vi "HEWH Write Standard Tests.vi"(8 "Error In":errorcluster, 11 "24HR Test - Standard":T1[](array[typedef])=[{"Sequence #"=1.0, "Cycles"=1, "Mode Setting"="", "Flow Rate (GPM)"=3.0, "Temperature (F)"=58.0, "Reset Timer"=FALSE, "Use Temp Decline Method"=FALSE, "Terminate Condition"=enum."C9-Do Nothing", "Condition Value #1"=0.0, "UE"=FALSE, "LE"=FALSE, "Comp"=FALSE, "Fan"=FALSE, "Test End Time (Sec)"=0.0, "Purge Until Cutout"=FALSE, "Start Conditions"=enum."Heat Source Cutout", "Condition Value #2"=0.0, "Remove Power"=FALSE, "Time"=82800.0, "Check Special Cond."=enum."SC1-Do Nothing", "Condition#"=enum."N/A", "Draw Flags"=enum."N/A", "Data Processing Delay (FHD 15sec, UEF 5 Sec)"=5.0, "Test Complete"=FALSE}, {"Sequence #"=2.0, "Cycles"=1, "Mode Setting"="", "Flow Rate (GPM)"=3.0, "Temperature (F)"=58.0, "Reset Timer"=TRUE, "Use Temp Decline Method"=TRUE, "Terminate Condition"=enum."C1-Terminate Draw @ Gallon Mark", "Condition Value #1"=10.72, "UE"=FALSE, "LE"=FALSE, "Comp"=FALSE, "Fan"=FALSE, "Test End Time (Sec)"=0.0, "Purge Until Cutout"=FALSE, "Start Conditions"=enum."At Time (Seconds)", "Condition Value #2"=0.0, "Remove Power"=FALSE, "Time"=82800.0, "Check Special Cond."=enum."SC1-Do Nothing", "Condition#"=enum."N/A", "Draw Flags"=enum."N/A", "Data Processing Delay (FHD 15sec, UEF 5 Sec)"=5.0, "Test Complete"=FALSE}, {"Sequence #"=3.0, "Cycles"=1, "Mode Setting"="", "Flow Rate (GPM)"=3.0, "Temperature (F)"=58.0, "Reset Timer"=FALSE, "Use Temp Decline Method"=FALSE, "Terminate Condition"=enum."C1-Terminate Draw @ Gallon Mark", "Condition Value #1"=10.72, "UE"=FALSE, "LE"=FALSE, "Comp"=FALSE, "Fan"=FALSE, "Test End Time (Sec)"=0.0, "Purge Until Cutout"=FALSE, "Start Conditions"=enum."At Time (Seconds)", "Condition Value #2"=3600.0, "Remove Power"=FALSE, "Time"=82800.0, "Check Special Cond."=enum."SC1-Do Nothing", "Condition#"=enum."N/A", "Draw Flags"=enum."N/A", "Data Processing Delay (FHD 15sec, UEF 5 Sec)"=5.0, "Test Complete"=FALSE}, {"Sequence #"=4.0, "Cycles"=1, "Mode Setting"="", "Flow Rate (GPM)"=3.0, "Temperature (F)"=58.0, "Reset Timer"=FALSE, "Use Temp Decline Method"=FALSE, "Terminate Condition"=enum."C1-Terminate Draw @ Gallon Mark", "Condition Value #1"=10.72, "UE"=FALSE, "LE"=FALSE, "Comp"=FALSE, "Fan"=FALSE, "Test End Time (Sec)"=0.0, "Purge Until Cutout"=FALSE, "Start Conditions"=enum."At Time (Seconds)", "Condition Value #2"=7200.0, "Remove Power"=FALSE, "Time"=82800.0, "Check Special Cond."=enum."SC1-Do Nothing", "Condition#"=enum."N/A", "Draw Flags"=enum."N/A", "Data Processing Delay (FHD 15sec, UEF 5 Sec)"=5.0, "Test Complete"=FALSE}, {"Sequence #"=5.0, "Cycles"=1, "Mode Setting"="", "Flow Rate (GPM)"=3.0, "Temperature (F)"=58.0, "Reset Timer"=FALSE, "Use Temp Decline Method"=FALSE, "Terminate Condition"=enum."C1-Terminate Draw @ Gallon Mark", "Condition Value #1"=10.72, "UE"=FALSE, "LE"=FALSE, "Comp"=FALSE, "Fan"=FALSE, "Test End Time (Sec)"=0.0, "Purge Until Cutout"=FALSE, "Start Conditions"=enum."At Time (Seconds)", "Condition Value #2"=10800.0, "Remove Power"=FALSE, "Time"=82800.0, "Check Special Cond."=enum."SC1-Do Nothing", "Condition#"=enum."N/A", "Draw Flags"=enum."N/A", "Data Processing Delay (FHD 15sec, UEF 5 Sec)"=5.0, "Test Complete"=FALSE}, {"Sequence #"=6.0, "Cycles"=1, "Mode Setting"="", "Flow Rate (GPM)"=3.0, "Temperature (F)"=58.0, "Reset Timer"=FALSE, "Use Temp Decline Method"=FALSE, "Terminate Condition"=enum."C1-Terminate Draw @ Gallon Mark", "Condition Value #1"=10.72, "UE"=FALSE, "LE"=FALSE, "Comp"=FALSE, "Fan"=FALSE, "Test End Time (Sec)"=0.0, "Purge Until Cutout"=FALSE, "Start Conditions"=enum."At Time (Seconds)", "Condition Value #2"=14400.0, "Remove Power"=FALSE, "Time"=82800.0, "Check Special Cond."=enum."SC1-Do Nothing", "Condition#"=enum."N/A", "Draw Flags"=enum."N/A", "Data Processing Delay (FHD 15sec, UEF 5 Sec)"=5.0, "Test Complete"=FALSE}, {"Sequence #"=7.0, "Cycles"=1, "Mode Setting"="", "Flow Rate (GPM)"=3.0, "Temperature (F)"=58.0, "Reset Timer"=FALSE, "Use Temp Decline Method"=FALSE, "Terminate Condition"=enum."C1-Terminate Draw @ Gallon Mark", "Condition Value #1"=10.72, "UE"=FALSE, "LE"=FALSE, "Comp"=FALSE, "Fan"=FALSE, "Test End Time (Sec)"=86400.0, "Purge Until Cutout"=FALSE, "Start Conditions"=enum."At Time (Seconds)", "Condition Value #2"=18000.0, "Remove Power"=TRUE, "Time"=82800.0, "Check Special Cond."=enum."SC1-Do Nothing", "Condition#"=enum."N/A", "Draw Flags"=enum."N/A", "Data Processing Delay (FHD 15sec, UEF 5 Sec)"=5.0, "Test Complete"=FALSE}] {"Time" format="%<%H:%M:%S>t"}) -> (0 "Error Out":errorcluster, 3 "Save String":string[][](array[string]))   [LabVIEW 2016]
uses:
  Type Definitions/PRAT Test.ctl
  Utility/Save File/File Setup (Public)/Type Definition/Save File HEWH Heating Control Mode.ctl
  Draw Water Specific/Type Definitions/Terminate Draw Conditions.ctl
  Type Definitions/HEWH Start Conditions.ctl
  Draw Water Specific/Type Definitions/Check Special Condtions.ctl
  Draw Water Specific/Type Definitions/HEWH Special Condition Check.ctl
  Type Definitions/HEWH Draw Flag ENUM.ctl
  <vilib>/Utility/file.llb/Write Delimited Spreadsheet (string).vi
  Utility/Save File/File Setup.lvlib
panel:
  in  "file path (dialog if empty)":path
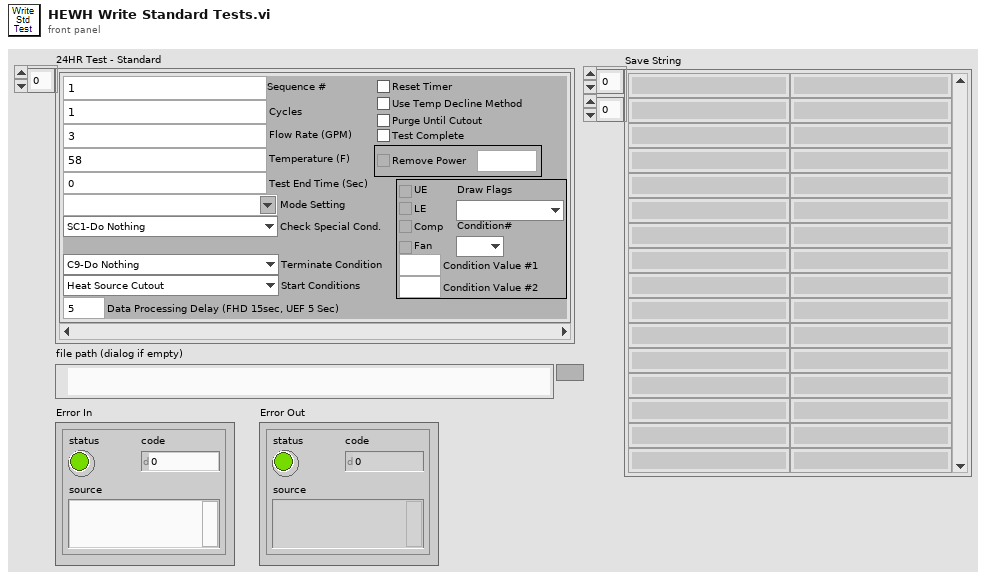
[diagram p1: front panel]
types:
  T1 = typedef "PRAT Test.ctl" = cluster{"Sequence #":dbl, "Cycles":i32, "Mode Setting":T2, "Flow Rate (GPM)":dbl, "Temperature (F)":dbl, "Reset Timer":bool, "Use Temp Decline Method":bool, "Terminate Condition":T3, "Condition Value #1":dbl, "UE":bool, "LE":bool, "Comp":bool, "Fan":bool, "Test End Time (Sec)":dbl, "Purge Until Cutout":bool, "Start Conditions":T4, "Condition Value #2":dbl, "Remove Power":bool, "Time":dbl, "Check Special Cond.":T5, "Condition#":T6, "Draw Flags":T7, "Data Processing Delay (FHD 15sec, UEF 5 Sec)":dbl, "Test Complete":bool}
  T2 = typedef "File Setup.lvlib/Save File HEWH Heating Control Mode.ctl" = string
  T3 = typedef "Terminate Draw Conditions.ctl" = enum16{"C1-Terminate Draw @ Gallon Mark", "C2-Special Last Draw (HU Test)", "C3-RTD Out <=", "C4-Mean Tank Temp <=", "C5-Decrease RTD Out (Deg F)", "C6-Time (Seconds)", "C7-Until Any Heat Source", "C8-Specific Heat Source", "C9-Do Nothing"}
  T4 = typedef "HEWH Start Conditions.ctl" = enum16{"Heat Source Cutout", "At Time (Seconds)", "Every X (Seconds)", "T2 >= X° Below Setpoint", "Seconds From Complete", "Wait for LE & Comp Cutout", "Wait for Comp Cutout", "Wait for LE Cutout", "Wait for UE Cutout"}
  T5 = typedef "Check Special Condtions.ctl" = enum16{"SC1-Do Nothing", "SC2-Check Heat Source (On-C2/Off-C1)", "SC3-Check Skip Condition", "SC4-Check Heat Source ON/Fail"}
  T6 = typedef "HEWH Special Condition Check.ctl" = enum16{"N/A", "C1", "C2", "Reset/Fail", "Skip Draw Sequence"}
  T7 = typedef "HEWH Draw Flag ENUM.ctl" = enum16{"N/A", "None(0)", "Sml(1)", "Med(2)", "SmlMed(3)", "Lrg(4)", "SmlLrg(5)", "MedLrg(6)", "SmlMedLrg(7)"}
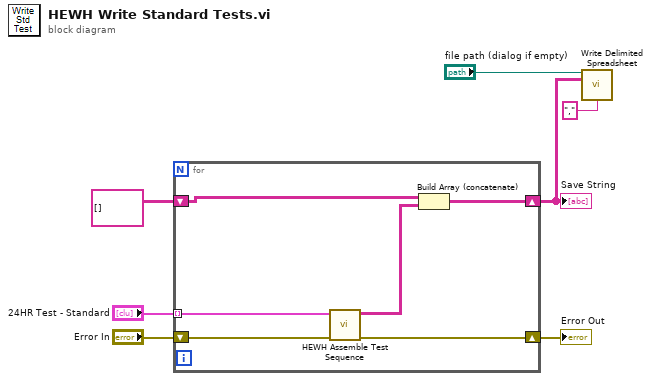
[diagram p0: block diagram]
diagram:
  n1 = for {
    tunnel: "24HR Test - Standard" -> [w13] mode=indexing
    shift-right: [w10] -> w3
    shift-left: string[][] [] -> [w12]
    shift-right: [w9] -> w5
    shift-left: "Error In" -> [w8]
    n2 = call "HEWH Assemble Test Sequence.vi"("Error In"=w8, "Cluster"=w13) -> ("Error Out"=w9:errorcluster, "String Test Seq"=w11:string[][])  [unwired: 8 in]
    n3 = Build Array (concatenate)(w12, w11) -> (w10:string[][])
  }
  "Save String" <- w3
  "Error Out" <- w5
  n4 = call-poly <vilib>:"Write Delimited Spreadsheet.vi"("file path (dialog if empty)"="file path (dialog if empty)", "2D data"=w3, "delimiter (\\t)"="," ("delimiter (\\t)")) -> ()  [unwired: 11 in, 2 out]
